vi "AcquisitionTestCompile.vi"() -> ()   [LabVIEW 2013]
doc: "This is the FPGA VI for the 10-Tap 8-Bit Camera with DRAM example. This example demonstrates how to acquire images from a 10-tap, 8-bit, extended configuration, Camera Link camera and transfer the images to the host. This example supports area scan and line scan cameras for both continuous and finite acquisitions.\n\nThis example also demonstrates the use of DRAM as a frame buffer for very high speed acquisitions. Data packing and flow-control are also employed to maximize use of the available DRAM and FIFOs in terms of both memory space and performance.\n\nAdditionally, the example demonstrates the serial server, which allows third-party camera configuration utilities to communicate with the camera using the Camera Link serial interface while this VI is running."
uses:
  <vilib>/rvi/DataTransferAndStorage/Container/XNode/niFpgaContainer.xnode
  <vilib>/Platform/TimedLoop/XDataNode/XDataNode.xnode
  <vilib>/Platform/TimedLoop/XDataNode/timing_clust.ctl
  <vilib>/Platform/TimedLoop/XDataNode/XDNodeRunTimeDep.lvlib
  <vilib>/Platform/TimedLoop/XDataNode/wakeup.ctl
  <vilib>/Platform/TimedLoop/XDataNode/nitl_modes.ctl
  <vilib>/eio/EIONode/EIONode.xnode
  <vilib>/rvi/eio/common/nirviEmuTemplateMethod_errors.vi
  <vilib>/rvi/FIFO/Fifo_Resource/nirvififoEmulationGetNumberOfElementsToRead.vi
  <vilib>/rvi/interface/RandomDataEmulation/nirviRandomDataFpgaReadWriteTemplate.vi
  <vilib>/rvi/FIFO/Fifo_Resource/nirvififoEmulationRead.vi
  <vilib>/rvi/FIFO/Fifo_Resource/nirvififoEmulationWrite.vi
  Common/CL Data to Pixels/10 Tap 8-Bit.vi
  FPGA/10-Tap Data/10-Tap Conversion Enum.ctl
  FPGA/Globals/Accumulated Sector Intensity.vi
  FPGA/Globals/Pixel Location Global.vi
  Common/CL Signal Mapping.ctl
  Common/CL Configuration.ctl
  FPGA/Sector/Background/Average Sector Background Intensity Cluster.ctl
  FPGA/Sector/Accumulate/Sector Parameter Cluster.ctl
panel:
  in  "# of Frames to Average":u8
  out "Average Background Sector":T1[](array[typedef])
  in  "Sector Parameters Right":T2={"Start Angle"=0.13543701171875, "End Angle"=0.30462646484375, "Inner Radius"=309, "Outter Radius"=405, "Hinge X"=1106, "Hinge Y"=803, "NumWingSectors"=8}
  in  "Sector Parameters Left":T2={"Start Angle"=0.6541748046875, "End Angle"=0.856201171875, "Inner Radius"=309, "Outter Radius"=405, "Hinge X"=947, "Hinge Y"=829, "NumWingSectors"=8}
  in  "Sim":bool=TRUE
  in  "CL Config.Configuration":T3=enum."Full"
  in  "CL Config.Signal Mapping":T4=enum."Basler 10-tap"
  in  "CL Config.Line Scan":bool
  in  "CL Config.DVAL Active High":bool=TRUE
  in  "CL Config.LVAL Active High":bool=TRUE
  in  "CL Config.FVAL Active High":bool=TRUE
  in  "CL Config.Spare Active High":bool=TRUE
  in  "Acq Control.Line Scan Height":u32
  in  "Acq Control.Frames To Acq":u32
  in  "Acq Control.Acquire":bool
  in  "Acq Control.Cancel Acq":bool
  in  "Acq Control.Ignore DVAL":bool
  in  "Acq Control.Initialize":bool
  out "Acq Status.Acq In Progress":bool
  out "Acq Status.Clocks Per Line":u32
  out "Acq Status.Frames Acq'd":u32
  out "Acq Status.Lines Per Frame":u32
  out "Acq Status.DMA Write Timeout":bool
  out "Acq Status.Initialized":bool
  in  "UART.Baud Rate":u8
  in  "UART.Transmit":bool
  in  "UART.Tx Data":u8[](array[numeric])=[0, 0, 0, 0, 0, 0, 0, 0, 0, 0] format="%02x"
  in  "UART.Set Baud Rate":bool
  in  "UART.Byte Mode":bool=TRUE
  out "UART.Rx Ready":bool
  out "UART.Break Indicator":bool
  out "UART.Framing Error":bool
  out "UART.Overrun Error":bool
  out "UART.Tx Ready":bool
  out "UART.Rx Data":u8 format="%02x"
  in  "UART.Receive":bool
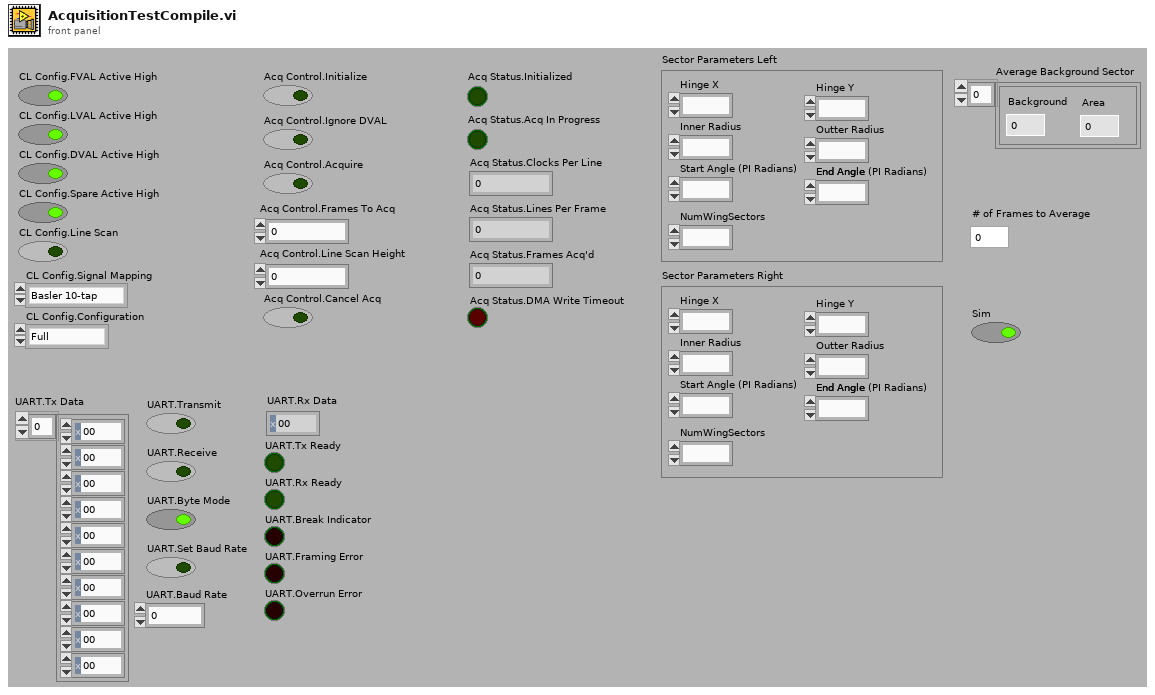
[diagram p1: front panel]
types:
  T1 = typedef "Average Sector Background Intensity Cluster.ctl" = cluster{"Background":u8, "Area":u16}
  T2 = typedef "Sector Parameter Cluster.ctl" = cluster{"Start Angle":fxp<+/-,17,2>, "End Angle":fxp<+,17,3>, "Inner Radius":u16, "Outter Radius":u16, "Hinge X":u16, "Hinge Y":u16, "NumWingSectors":u8}
  T3 = typedef "CL Configuration.ctl" = enum8{"Base", "Medium", "Full"}
  T4 = typedef "CL Signal Mapping.ctl" = enum8{"Standard", "Basler 10-tap", "Vosskühler 10-tap"}
  T5 = typedef "XDNodeRunTimeDep.lvlib/timing_clust.ctl" = cluster{"Expected End [f-1]":u64, "Actual End [f-1]":u64, "Finished Late? [f-1]":bool, "Expected End [i-1]":u64, "Actual End [i-1]":u64, "Finished Late? [i-1]":bool, "Expected Start [i]":u64, "Actual Start [i]":u64, "Expected Start [f]":u64, "Actual Start [f]":u64, "Source Name":string, "Structure Name":string, "Period":i64, "Deadline":i64, "Offset":i64, "Start":i64, "Priority":i32, "Timeout":i32, "Mode":T6, "Wakeup Reason":T7, "Error":errorcluster, "Source Type":string, "Secondary Source Type":string, "Global End Time":u64, "Global Start Time":u64, "Frame Duration":u64, "Iteration Duration":u64, "Assigned CPU":i32, "I/O Scan Engine Mode":u32}
  T6 = typedef "XDNodeRunTimeDep.lvlib/nitl_modes.ctl" = enum32{"No Change", "Process missed periods, maintain original phase", "Discard missed periods, maintain original phase", "Process missed periods, ignore original phase", "Discard missed periods, ignore original phase"}
  T7 = typedef "XDNodeRunTimeDep.lvlib/wakeup.ctl" = enum32{"Normal", "Aborted", "Asynchronous wakeup", "Timing source error", "Timed loop error", "Timeout"}
  T8 = typedef "10-Tap Conversion Enum.ctl" = enum16{"10-Tap to 16 and 64", "16 and 64 to 10-Tap"}
  T9 = cluster{"Enables Valid":bool, "Frame Valid":bool, "Line Valid":bool, "Data Valid":bool}
  T10 = typedef "10-Tap 8-bit Cluster.ctl" = cluster{"Pixel 0":u8, "Pixel 1":u8, "Pixel 2":u8, "Pixel 3":u8, "Pixel 4":u8, "Pixel 5":u8, "Pixel 6":u8, "Pixel 7":u8, "Pixel 8":u8, "Pixel 9":u8}
  T11 = cluster{"Tx Data":u8[], "Transmit":bool, "Receive":bool, "Byte Mode":bool, "Set Baud Rate":bool, "Baud Rate":u8}
  T12 = cluster{"Rx Data":u8, "Turn Off Transmit":bool, "Turn Off Receive":bool, "Turn Off Set Baud Rate":bool, "Tx Ready":bool, "Rx Ready":bool, "Break Indicator":bool, "Framing Error":bool, "Overrun Error":bool}
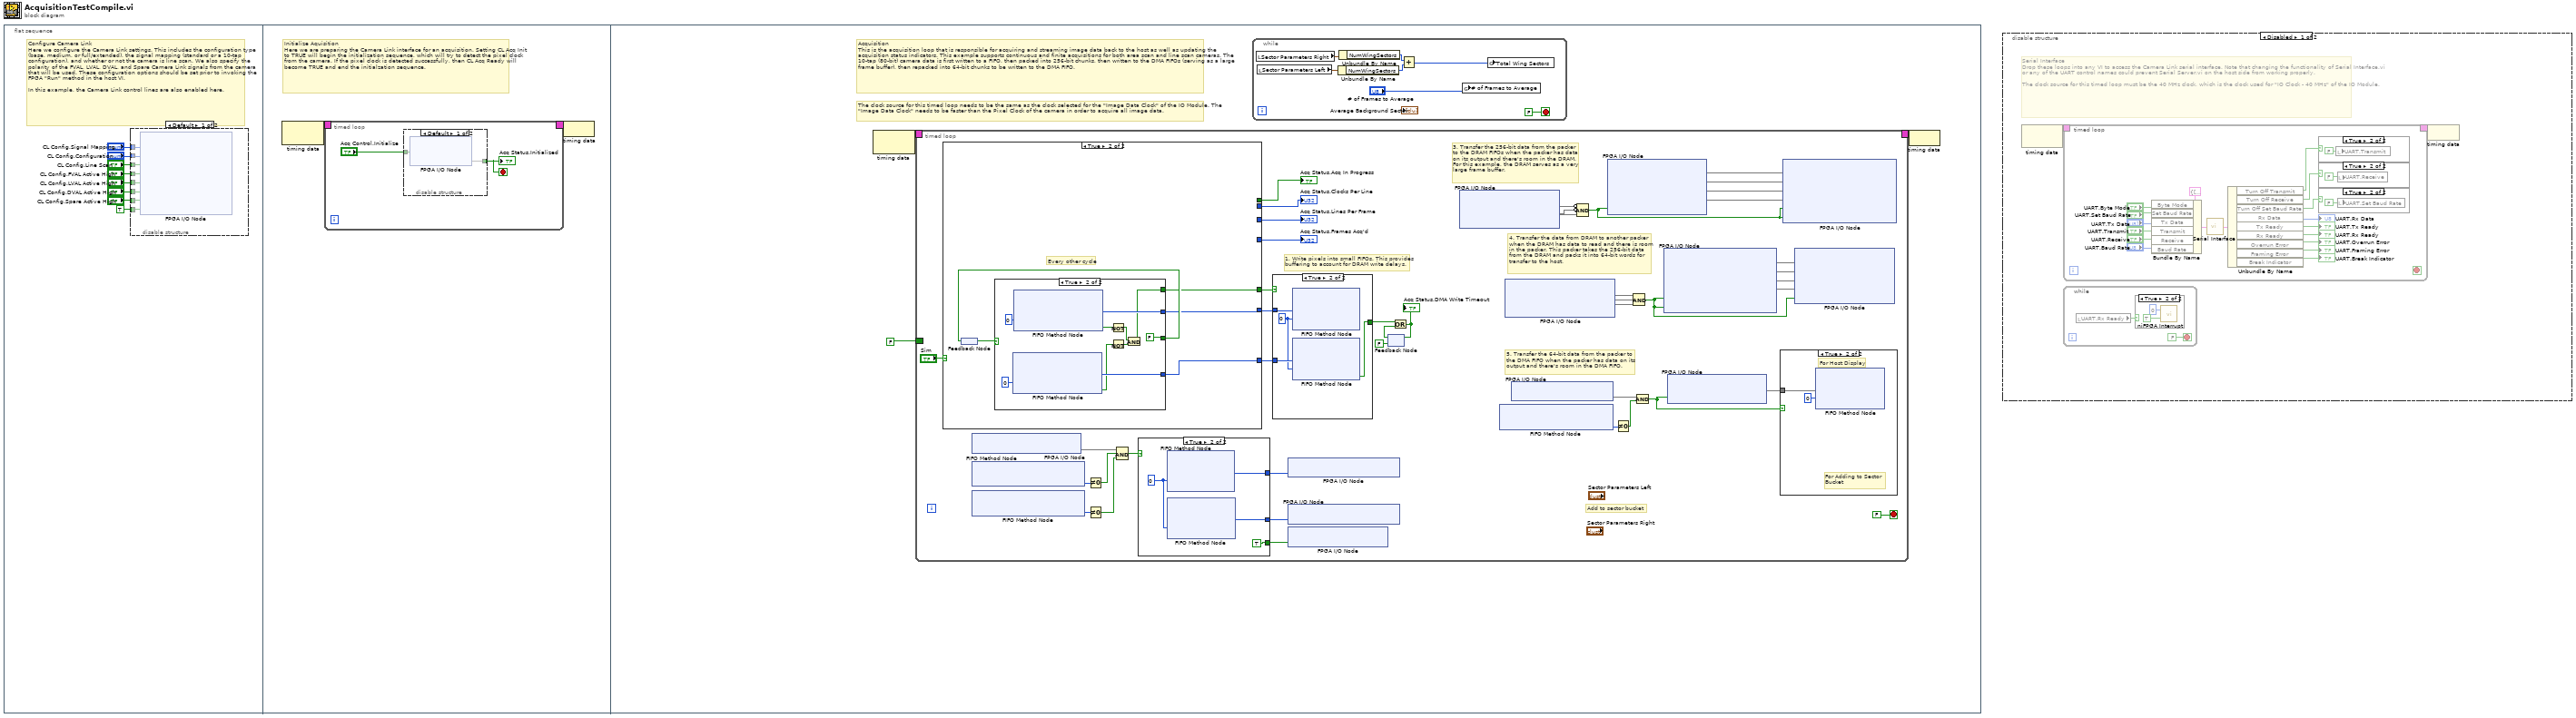
[diagram p0: block diagram]
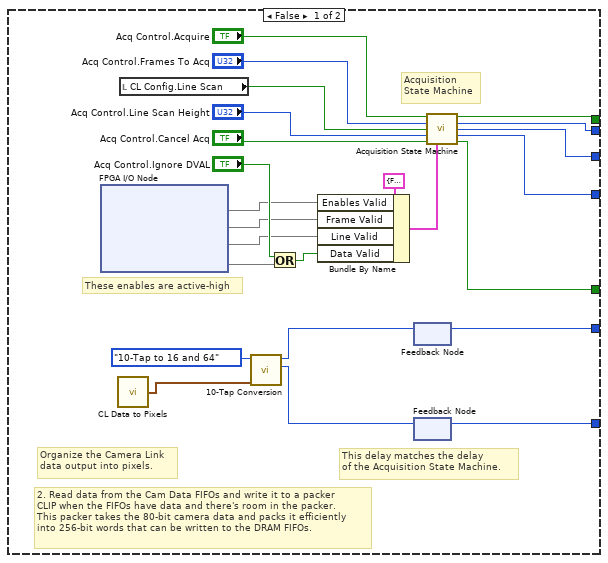
[diagram p10: hidden frame]
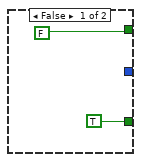
[diagram p11: hidden frame]
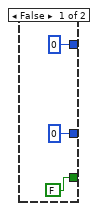
[diagram p12: hidden frame]
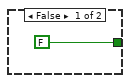
[diagram p13: hidden frame]
diagram:
  n1 = flat-sequence {
    frame #0 {
      # "Configure Camera Link\nHere we configure the Camera Link settings. This includes the configuration type (base, medium, or full/extended), the signal mapping (standard or a 10-tap configuration), and whether or not the camera is line scan. We also specify the polarity of the FVAL, LVAL, DVAL, and Spare Camera Link signals from the camera that will be used. These configuration options should be set prior to invoking the FPGA \"Run\" method in the host VI.\n\nIn this example, the Camera Link control lines are also enabled here."
      n2 = disable-structure shown="Default" {
        disable-tunnel: "CL Config.FVAL Active High" -> [w16 _]
        disable-tunnel: "CL Config.LVAL Active High" -> [w15 _]
        disable-tunnel: "CL Config.DVAL Active High" -> [w14 _]
        disable-tunnel: "CL Config.Spare Active High" -> [w13 _]
        disable-tunnel: "CL Config.Signal Mapping" -> [w12 _]
        disable-tunnel: "CL Config.Configuration" -> [w11 _]
        disable-tunnel: "CL Config.Line Scan" -> [w10 _]
        disable-tunnel: TRUE ("IO Module\\CL Control Enable") -> [w9 _]
        frame condition #0 {
          n3 = xnode "FPGA I/O Node"("CL Set Signal Mapping"=w12, "CL Set Configuration"=w11, "CL Set Line Scan"=w10, "CL Set FVAL Active High"=w16, "CL Set LVAL Active High"=w15, "CL Set DVAL Active High"=w14, "CL Set Spare Active High"=w13, "CL Control Enable"=w9) -> ()  [unwired: 8 in, 8 out]
        }
        frame condition #1 (active) {
        }
      }
    }
    frame #1 {
      # "Initialize Aquisition\nHere we are preparing the Camera Link interface for an acquisition. Setting CL Acq Init to TRUE will begin the initialization sequence, which will try to detect the pixel clock from the camera. If the pixel clock is detected successfully, then CL Acq Ready will become TRUE and end the initialzation sequence."
      n4 = node-c288() -> (w18:T5)  [unwired: 1 out]
      n5 = timed-loop {
        timing: w18 -> [_]
        timing-out: [_] -> w17
        stop <- w19 stop-if-true
        n6 = disable-structure shown="Default" {
          disable-tunnel: "Acq Control.Initialize" -> [w22 w23]
          disable-tunnel: [w21 w23] -> w19
          frame condition #0 {
            n7 = xnode "FPGA I/O Node"("CL Acq Init"=w22) -> ("CL Acq Ready"=w21)  [unwired: 2 in, 2 out]
          }
          frame condition #1 (active) {
          }
        }
        "Acq Status.Initialized" <- w19
      }
      n8 = node-c288(w17) -> ()
    }
    frame #2 {
      # "The clock source for this timed loop needs to be the same as the clock selected for the \"Image Data Clock\" of the IO Module. The \"Image Data Clock\" needs to be faster than the Pixel Clock of the camera in order to acquire all image data."
      # "Acquisition\nThis is the acquisition loop that is responsible for acquiring and streaming image data back to the host as well as updating the acquisition status indicators. This example supports continuous and finite acquisitions for both area scan and line scan cameras. The 10-tap (80-bit) camera data is first written to a FIFO, then packed into 256-bit chunks, then written to the DMA FIFOs (serving as a large frame buffer), then repacked into 64-bit chunks to be written to the DMA FIFO."
      n9 = node-c288() -> (w30:T5)  [unwired: 1 in]
      n10 = timed-loop {
        timing: w30 -> [_]
        timing-out: [_] -> w29
        border: FALSE -> [_]
        stop <- FALSE stop-if-true
        # "Add to sector bucket"
        # "5. Transfer the 64-bit data from the packer to\nthe DMA FIFO when the packer has data on its\noutput and there's room in the DMA FIFO."
        # "4. Transfer the data from DRAM to another packer\nwhen the DRAM has data to read and there is room\nin the packer. This packer takes the 256-bit data\nfrom the DRAM and packs it into 64-bit words for\ntransfer to the host."
        # "3. Transfer the 256-bit data from the packer\nto the DRAM FIFOs when the packer has data\non its output and there's room in the DRAM.\nFor this example, the DRAM serves as a very\nlarge frame buffer."
        # "1. Write pixels into small FIFOs. This provides\nbuffering to account for DRAM write delays."
        n11 = case shown="True" "Sim" {
          tunnel: [w105 w106] -> w79
          tunnel: [w104 w107] -> w74
          tunnel: [w86 w109] -> w62
          tunnel: [w90 _] -> w61
          tunnel: [w89 _] -> w60
          tunnel: [w88 _] -> w59
          tunnel: [w87 _] -> w58
          frame False {
            # "These enables are active-high"
            # "Acquisition\nState Machine"
            # "2. Read data from the Cam Data FIFOs and write it to a packer\nCLIP when the FIFOs have data and there's room in the packer.\nThis packer takes the 80-bit camera data and packs it efficiently\ninto 256-bit words that can be written to the DRAM FIFOs."
            # "Organize the Camera Link\ndata output into pixels."
            # "This delay matches the delay\nof the Acquisition State Machine."
            n12 = xnode "FPGA I/O Node"() -> ("CL Output Valid"=w94, "CL Frame Valid"=w95, "CL Line Valid"=w96, "CL Data Valid"=w99)  [unwired: 4 in, 4 out]
            n13 = call-poly "CL Data to Pixels.vi"() -> ("Pixels"=w82:T10)  [unwired: 1 in]
            n14 = local read "CL Config.Line Scan"() -> (w102:bool)
            n15 = call "10-Tap Conversion.vi"("10 Tap In"=w82, "Operation"=10-Tap_Conversion_Enum."10-Tap to 16 and 64") -> ("64 Bit Out"=w83:u64, "16 Bit Out"=w84:u16)  [unwired: 7 in, 1 out]
            n16 = Or(x="Acq Control.Ignore DVAL", y=w99) -> (x .or. y?=w100:bool)
            n17 = Bundle By Name(cluster=T9 {"Enables Valid"=FALSE, "Frame Valid"=FALSE, "Line Valid"=FALSE, "Data Valid"=FALSE} ("Enables"), "Enables Valid"=w94, "Frame Valid"=w95, "Line Valid"=w96, "Data Valid"=w100) -> (w97:T9)
            n18 = feedback #1() -> (w104:u16)  [unwired: 1 in]
            n19 = feedback-in #1(w84) -> ()
            n20 = feedback #2() -> (w105:u64)  [unwired: 1 in]
            n21 = feedback-in #2(w83) -> ()
            n22 = call "Acquisition State Machine.vi"("Acquire"="Acq Control.Acquire", "Frames to Acquire"="Acq Control.Frames To Acq", "Line Scan"=w102, "Line Scan Height"="Acq Control.Line Scan Height", "Cancel Acq"="Acq Control.Cancel Acq", "Enables"=w97) -> ("Acq In Progress"=w90:bool, "Num Clocks Per Line"=w89:u32, "Num Lines Per Frame"=w88:u32, "Num Frames Acq'd"=w87:u32, "Capture Cycle"=w86:bool)  [unwired: 4 in, 1 out]
          }
          frame True {
            # "Every other cycle"
            n23 = feedback #3() -> (w108:bool)
            n24 = case shown="True" w108 {
              tunnel: [_ w122] -> w107
              tunnel: [_ w121] -> w106
              tunnel: [FALSE w114] -> w109
              tunnel: [TRUE FALSE] -> w110
              frame False {
              }
              frame True {
                n25 = xnode ("FIFO Method Node")("Timeout"=0) -> ("Element"=w121:u64, "Timed Out?"=w117:bool)  [unwired: 1 in, 1 out]
                n26 = xnode ("FIFO Method Node")("Timeout"=0) -> ("Element"=w122:u16, "Timed Out?"=w118:bool)  [unwired: 1 in, 1 out]
                n27 = Not(x=w118) -> (.not. x?=w116:bool)
                n28 = Not(x=w117) -> (.not. x?=w115:bool)
                n29 = And(x=w116, y=w115) -> (x .and. y?=w114:bool)
              }
            }
            n30 = feedback-in #3(w110) -> ()
          }
        }
        "Acq Status.Frames Acq'd" <- w58
        "Acq Status.Lines Per Frame" <- w59
        "Acq Status.Clocks Per Line" <- w60
        "Acq Status.Acq In Progress" <- w61
        n31 = xnode "FPGA I/O Node"() -> ("Pack 80 to 256\\Ready For Write"=w68)  [unwired: 1 in, 1 out]
        n32 = xnode ("FIFO Method Node")() -> ("Number of Elements to Read"=w72:u32)  [unwired: 1 in, 1 out]
        n33 = xnode ("FIFO Method Node")() -> ("Number of Elements to Read"=w71:u32)  [unwired: 1 in, 1 out]
        n34 = Not Equal To 0?(x=w72) -> (x != 0?=w66:bool)
        n35 = Not Equal To 0?(x=w71) -> (x != 0?=w65:bool)
        n36 = Compound Arithmetic op=AND(w68, w66, w65) -> (w67:bool)
        n37 = case shown="True" w67 {
          tunnel: [u16 0 ("Element") w129] -> w73
          tunnel: [u64 0 ("Element") w128] -> w69
          tunnel: [FALSE TRUE] -> w70
          frame False {
          }
          frame True {
            w127 = 0 ("Timeout")
            n38 = xnode ("FIFO Method Node")("Timeout"=w127) -> ("Element"=w129:u16)  [unwired: 1 in, 2 out]
            n39 = xnode ("FIFO Method Node")("Timeout"=w127) -> ("Element"=w128:u64)  [unwired: 1 in, 2 out]
          }
        }
        n40 = case shown="True" w62 {
          tunnel: [FALSE ("Timed Out?") w133] -> w77
          tunnel: w79 -> [_ w134]
          tunnel: w74 -> [_ w132]
          frame False {
          }
          frame True {
            w131 = 0 ("Timeout")
            n41 = xnode ("FIFO Method Node")("Element"=w132, "Timeout"=w131) -> ()  [unwired: 1 in, 2 out]
            n42 = xnode ("FIFO Method Node")("Element"=w134, "Timeout"=w131) -> ("Timed Out?"=w133:bool)  [unwired: 1 in, 1 out]
          }
        }
        n43 = xnode "FPGA I/O Node"("Pack 80 to 256\\Data In Upper 16"=w73) -> ()  [unwired: 1 in, 1 out]
        n44 = xnode "FPGA I/O Node"("Pack 80 to 256\\Data In Lower 64"=w69) -> ()  [unwired: 1 in, 1 out]
        n45 = xnode "FPGA I/O Node"("Pack 80 to 256\\Write Enable"=w70) -> ()  [unwired: 1 in, 1 out]
        n46 = feedback #4(FALSE) -> (w76:bool)
        n47 = Or(x=w77, y=w76) -> (x .or. y?=w75:bool)
        "Acq Status.DMA Write Timeout" <- w75
        n48 = feedback-in #4(w75) -> ()
        n49 = xnode "FPGA I/O Node"() -> ("DRAM Bank 0\\Full"=w38, "Pack 80 to 256\\Output Valid"=w57)  [unwired: 3 in, 4 out]
        n50 = xnode ("FIFO Method Node")() -> ("Number of Elements to Write"=w40:u32)  [unwired: 1 in, 1 out]
        n51 = xnode "FPGA I/O Node"() -> ("DRAM Bank 1\\Data_Available"=w51, "DRAM Bank 0\\Data_Available"=w49, "Pack 256 To 64\\Ready for Write"=w50)  [unwired: 3 in, 3 out]
        n52 = xnode "FPGA I/O Node"() -> ("Pack 256 To 64\\Output Valid"=w42)  [unwired: 1 in, 1 out]
        n53 = Compound Arithmetic op=AND(invert w38, invert w38, w57) -> (w52:bool)
        n54 = xnode "FPGA I/O Node"("Pack 80 to 256\\Read Enable"=w52) -> ("Pack 80 To 256\\Data Out 3"=w56, "Pack 80 To 256\\Data Out 2"=w55, "Pack 80 To 256\\Data Out 1"=w54, "Pack 80 To 256\\Data Out 0"=w53)  [unwired: 5 in, 5 out]
        n55 = Not Equal To 0?(x=w40) -> (x != 0?=w41:bool)
        n56 = Compound Arithmetic op=AND(w51, w49, w50) -> (w44:bool)
        n57 = Compound Arithmetic op=AND(w42, w41) -> (w39:bool)
        n58 = xnode "FPGA I/O Node"("DRAM Bank 1\\Read"=w44, "DRAM Bank 0\\Read"=w44) -> ("DRAM Bank 1\\Read_Data_Upper"=w48, "DRAM Bank 1\\Read_Data_Lower"=w47, "DRAM Bank 0\\Read_Data_Upper"=w46, "DRAM Bank 0\\Read_Data_Lower"=w45)  [unwired: 6 in, 6 out]
        n59 = xnode "FPGA I/O Node"("Pack 256 to 64\\Read Enable"=w39) -> ("Pack 256 To 64\\Data Out 64"=w43)  [unwired: 2 in, 2 out]
        n60 = case shown="True" w39 {
          tunnel: w43 -> [_ w80]
          frame False {
          }
          frame True {
            # "For Adding to Sector \nBucket"
            # "For Host Display"
            n61 = xnode ("FIFO Method Node")("Element"=w80, "Timeout"=0) -> ()  [unwired: 1 in, 2 out]
          }
        }
        n62 = xnode "FPGA I/O Node"("DRAM Bank 1\\Write_Data_Upper"=w56, "DRAM Bank 1\\Write_Data_Lower"=w55, "DRAM Bank 0\\Write_Data_Upper"=w54, "DRAM Bank 0\\Write_Data_Lower"=w53, "DRAM Bank 1\\Write"=w52, "DRAM Bank 0\\Write"=w52) -> ()  [unwired: 6 in, 6 out]
        n63 = xnode "FPGA I/O Node"("Pack 256 To 64\\Data In 3"=w48, "Pack 256 To 64\\Data In 2"=w47, "Pack 256 To 64\\Data In 1"=w46, "Pack 256 To 64\\Data In 0"=w45, "Pack 256 to 64\\Write Enable"=w44) -> ()  [unwired: 5 in, 5 out]
      }
      n64 = while {
        stop <- FALSE stop-if-true
        n65 = local read "Sector Parameters Right"() -> (w36:T2)
        n66 = local read "Sector Parameters Left"() -> (w35:T2)
        n67 = Unbundle By Name(w35) -> ("NumWingSectors"=w33:u8)
        n68 = Unbundle By Name(w36) -> ("NumWingSectors"=w34:u8)
        n69 = Add(x=w34, y=w33) -> (x+y=w32:u8)
        n70 = global write "Pixel Location Global.vi" "# of Frames to Average"("# of Frames to Average") -> ()
        n71 = global write "Accumulated Sector Intensity.vi" "Total Wing Sectors"(w32) -> ()
      }
      n72 = node-c288(w29) -> ()
    }
  }
  n73 = disable-structure shown="Disabled" {
    frame Disabled {
      # "Serial Interface\nDrop these loops into any VI to access the Camera Link serial interface. Note that changing the functionality of Serial Interface.vi or any of the UART control names could prevent Serial Server.vi on the host side from working properly.\n\nThe clock source for this timed loop must be the 40 MHz clock, which is the clock used for \"IO Clock - 40 MHz\" of the IO Module."
      n74 = node-c288() -> (w140:T5)  [unwired: 1 out]
      n75 = timed-loop {
        timing: w140 -> [_]
        timing-out: [_] -> w139
        stop <- _ stop-if-true
        n76 = Bundle By Name(cluster=T11 {"Tx Data"=[0, 0, 0, 0, 0, 0, 0, 0, 0, 0], "Transmit"=FALSE, "Receive"=FALSE, "Byte Mode"=TRUE, "Set Baud Rate"=FALSE, "Baud Rate"=0} ("UART Inputs"), "Byte Mode"="UART.Byte Mode", "Set Baud Rate"="UART.Set Baud Rate", "Tx Data"="UART.Tx Data", "Transmit"="UART.Transmit", "Receive"="UART.Receive", "Baud Rate"="UART.Baud Rate") -> (w145:T11)
        n77 = call "Serial Interface.vi"("UART Inputs"=w145) -> ("UART Outputs"=w157:T12)
        n78 = Unbundle By Name(w157) -> ("Turn Off Transmit"=w150:bool, "Turn Off Receive"=w151:bool, "Turn Off Set Baud Rate"=w147:bool, "Rx Data"=→"UART.Rx Data":u8, "Tx Ready"=→"UART.Tx Ready":bool, "Rx Ready"=→"UART.Rx Ready":bool, "Overrun Error"=→"UART.Overrun Error":bool, "Framing Error"=→"UART.Framing Error":bool, "Break Indicator"=→"UART.Break Indicator":bool)
        n79 = case shown="True" w150 {
          frame False {
          }
          frame True {
            n80 = local write "UART.Transmit"(FALSE ("UART.Transmit")) -> ()
          }
        }
        n81 = case shown="True" w151 {
          frame False {
          }
          frame True {
            n82 = local write "UART.Receive"(FALSE ("UART.Receive")) -> ()
          }
        }
        n83 = case shown="True" w147 {
          frame False {
          }
          frame True {
            n84 = local write "UART.Set Baud Rate"(FALSE ("UART.Receive")) -> ()
          }
        }
      }
      n85 = while {
        stop <- FALSE stop-if-true
        n86 = local read "UART.Rx Ready"() -> (w142:bool)
        n87 = case shown="True" w142 {
          frame False {
          }
          frame True {
            n88 = call <vilib>:"niFPGA Interrupt.vi"("Wait Until Cleared (F)"=TRUE ("Wait Until Cleared"), "IRQ Number (0)"=u8 0 ("IRQ Number")) -> ()  [unwired: 1 in]
          }
        }
      }
      n89 = node-c288(w139) -> ()
    }
    frame Enabled {
    }
  }
